vi "Generate ConfigFile Path.vi"() -> (0 "ConfigFile path":path)   [LabVIEW 2020, in "FPGA Addon DMA Channels Interleaved System Tests.lvclass"]
uses:
  FPGA Addon DMA Channels Interleaved System Tests.lvclass
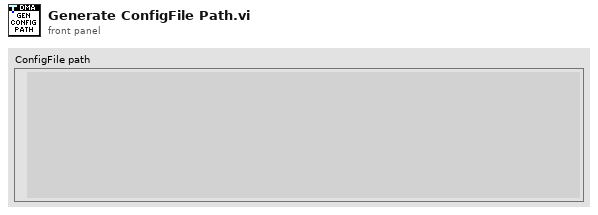
[diagram p1: front panel]
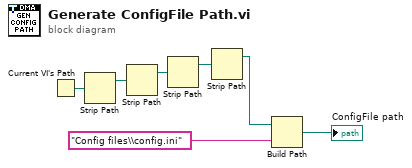
[diagram p0: block diagram]
diagram:
  n1 = Current VI's Path() -> (path=w7:path)
  n2 = Strip Path(path=w7) -> (stripped path=w6:path)  [unwired: 1 out]
  n3 = Strip Path(path=w6) -> (stripped path=w5:path)  [unwired: 1 out]
  n4 = Strip Path(path=w5) -> (stripped path=w4:path)  [unwired: 1 out]
  n5 = Strip Path(path=w4) -> (stripped path=w3:path)  [unwired: 1 out]
  n6 = Build Path(base path=w3, name or relative path="Config files\\config.ini") -> (appended path=→"ConfigFile path":path)
